vi "Initialize Hardware References.vi"(8 "error in (no error)":T3 caption="entrée d'erreur (pas d'erreur)", 11 "Ressources matérielles en entrée":T1) -> (0 "error out":T3 caption="sortie d'erreur", 3 "Ressources matérielles en sortie":T1)   [LabVIEW 2018, in "Acquisition.lvlib"]
doc: "Initialiser les références au matériel."
uses:
  Acquisition.lvlib
  Hardware Configuration.ctl
  Signal Type.ctl
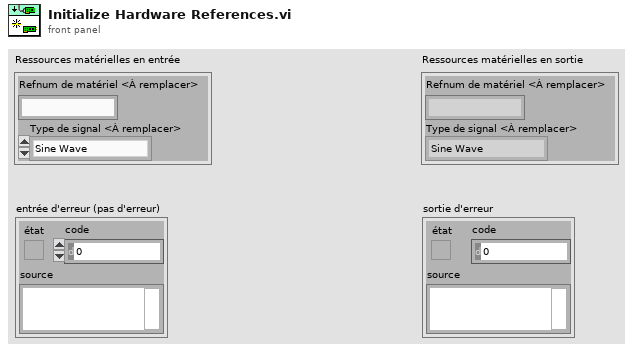
[diagram p1: front panel]
types:
  T1 = typedef "Acquisition.lvlib/Hardware Configuration.ctl" = cluster{"Refnum de matériel <À remplacer>":string, "Type de signal <À remplacer>":T2}
  T2 = typedef "Acquisition.lvlib/Signal Type.ctl" = enum16{"Sine Wave", "Square with Noise", "Signal triangulaire", "Simulation DAQ"}
  T3 = cluster{"état":bool, "code":i32, "source":string}
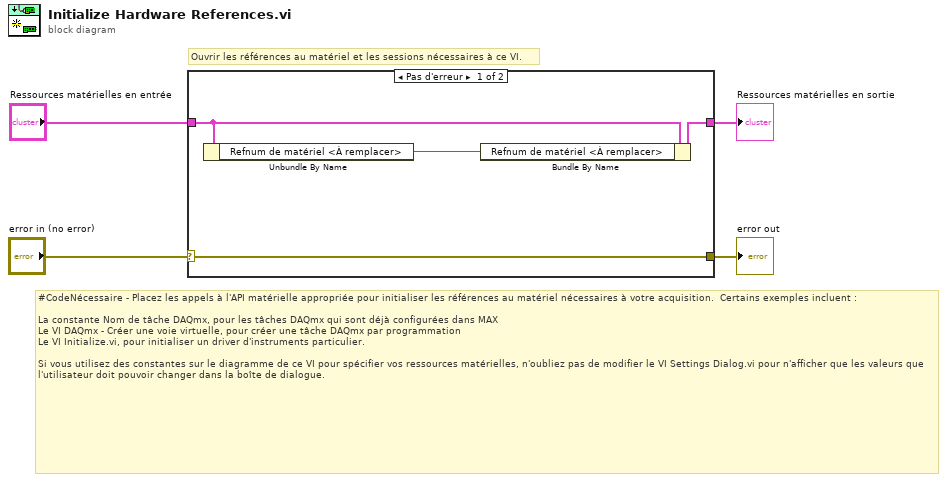
[diagram p0: block diagram]
diagram:
  # "Ouvrir les références au matériel et les sessions nécessaires à ce VI."
  # "#CodeNécessaire - Placez les appels à l'API matérielle appropriée pour initialiser les références au matériel nécessaires à votre acquisition.  Certains exemples incluent :\n\nLa constante Nom de tâche DAQmx, pour les tâches DAQmx qui sont déjà configurées dans MAX\nLe VI DAQmx - Créer une voie virtuelle, pour créer une tâche DAQmx par programmation\nLe VI Initialize.vi, pour initialiser un driver d'instruments particulier.\n\nSi vous utilisez des constantes sur le diagramme de ce VI pour spécifier vos ressources matérielles, n'oubliez pas de modifier le VI Settings Dialog.vi pour n'afficher que les valeurs que l'utilisateur doit pouvoir changer dans la boîte de dialogue."
  n1 = case shown="Pas d'erreur" "error in (no error)" {
    selector: "error in (no error)" -> [w7 w9]
    tunnel: [w7 w9] -> w3
    tunnel: "Ressources matérielles en entrée" -> [w6 w10]
    tunnel: [w8 w10] -> w1
    frame No Error {
      n2 = Unbundle By Name(w6) -> ("Refnum de matériel <À remplacer>"=w5:string)
      n3 = Bundle By Name(cluster=w6, "Refnum de matériel <À remplacer>"=w5) -> (w8:T1)
    }
    frame Error {
    }
  }
  "Ressources matérielles en sortie" <- w1
  "error out" <- w3
